vi "PAM icListen CC AV.vi"(4 "TCP IDs In":T2, 5 "Acq In":T1, 6 "icListen #":i32=1, 7 "Enabled":bool) -> (0 "TCP IDs Out":T2, 1 "Acq Out":T1, 3 "Stop":bool)   [LabVIEW 2020]
uses:
  icListen 1 Reset.vi
  icListen 1 Initialized.vi
  icListen 1 Connected.vi
  icListen 2 Reset.vi
  icListen 2 Initialized.vi
  icListen 2 Connected.vi
  icListen 3 Reset.vi
  icListen 3 Initialized.vi
  icListen 3 Connected.vi
  icListen 4 Reset.vi
  icListen 4 Initialized.vi
  icListen 4 Connected.vi
  icListen 1 Synchronization.vi
  icListen 1 Response.vi
  icListen 1 Metadata.vi
  icListen 2 Synchronization.vi
  icListen 2 Response.vi
  icListen 2 Metadata.vi
  icListen 3 Synchronization.vi
  icListen 3 Response.vi
  icListen 3 Metadata.vi
  icListen 4 Synchronization.vi
  icListen 4 Response.vi
  icListen 4 Metadata.vi
  PAM Array Buffer Size.vi
  icListen 1 Saving.vi
  icListen 2 Saving.vi
  icListen 3 Saving.vi
  icListen 4 Saving.vi
  icListen 1 Serial Number.vi
  icListen 2 Serial Number.vi
  icListen 3 Serial Number.vi
  icListen 4 Serial Number.vi
  PAM Library.lvlib
panel:
  out "Error Out":errorcluster
  out "Error Out":errorcluster
  out "Error Out":errorcluster
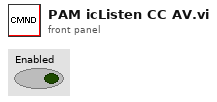
[diagram p1: front panel]
types:
  T1 = cluster{"State":enum16{"Align with Stream", "Read Header Byte", "Read Data Header", "Read Event Header", "Read Notification", "Read Data"}, "Sample Count":i32, "Timestamp":u64, "Payload":u16, "Repeated Error":i32, "Header Byte":string}
  T2 = cluster{"CC Id":refnum<k5>, "Waveform ID":refnum<k5>, "Spectrum ID":refnum<k5>, "Other Data ID":refnum<k5>}
  T3 = cluster{"System Time Status":u8, "Sync Status":u8, "PPS Count":u32, "Sync Offset":u32}
  T4 = cluster{"Date":string, "Time":string, "Temperature":dbl, "Humidity":dbl, "Battery Charge":i32}
  T5 = cluster{"default (0 U32) 2":i16, "default (0 U32)":i32, "unsigned 64bit integer":u64}
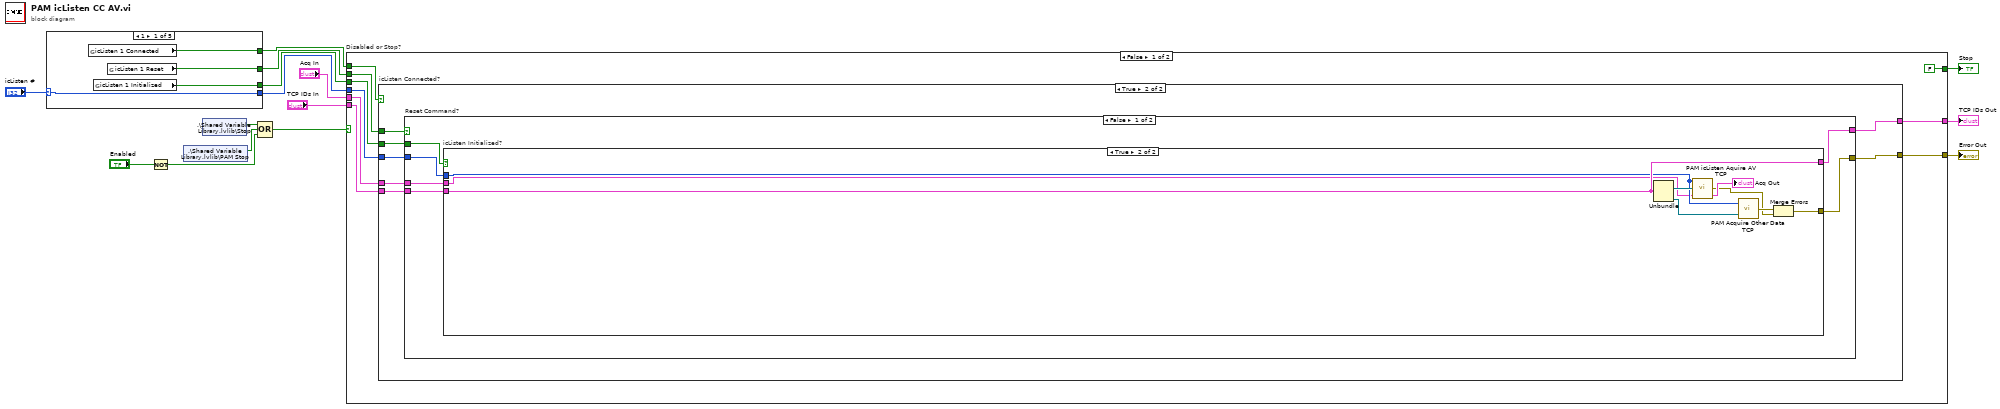
[diagram p0: block diagram]
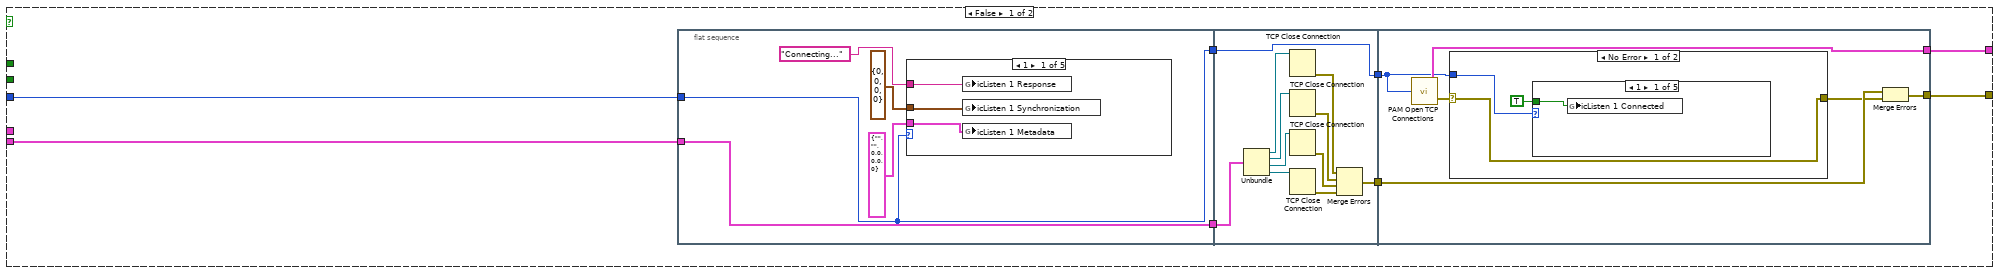
[diagram p2: hidden frame]
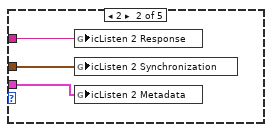
[diagram p3: hidden frame]
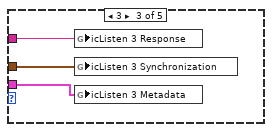
[diagram p4: hidden frame]
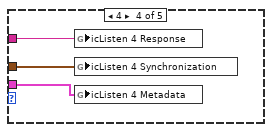
[diagram p5: hidden frame]
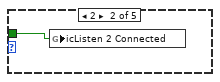
[diagram p7: hidden frame]
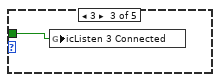
[diagram p8: hidden frame]
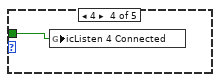
[diagram p9: hidden frame]
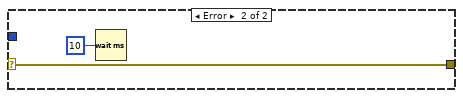
[diagram p11: hidden frame]
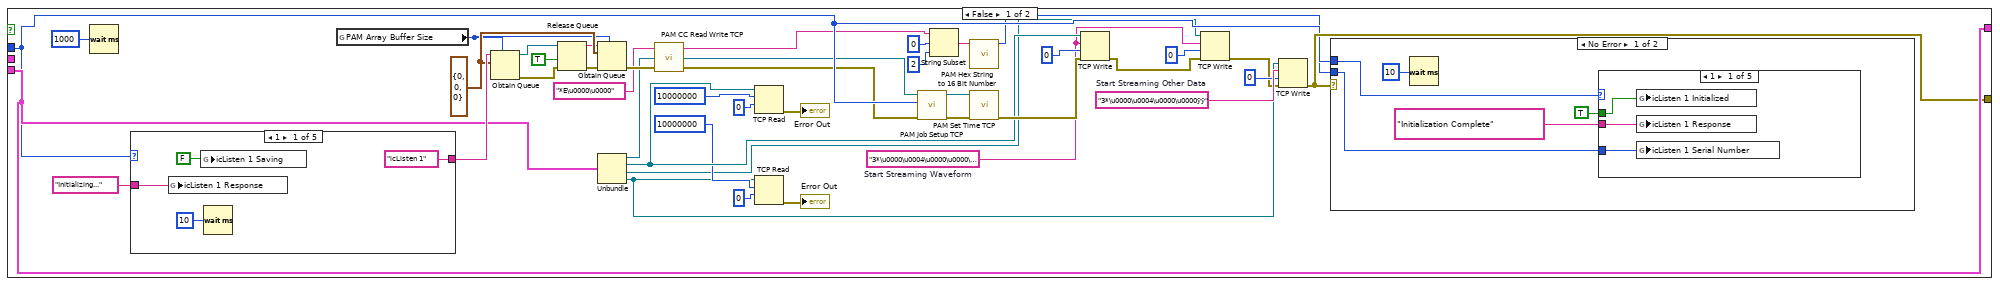
[diagram p12: hidden frame]
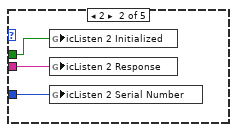
[diagram p13: hidden frame]
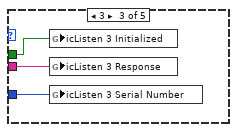
[diagram p14: hidden frame]
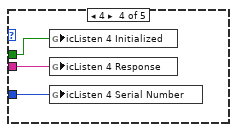
[diagram p15: hidden frame]
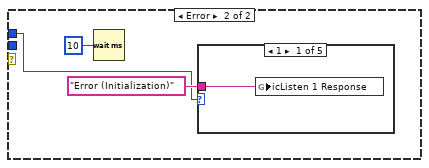
[diagram p17: hidden frame]
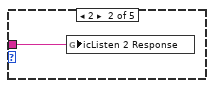
[diagram p18: hidden frame]
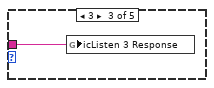
[diagram p19: hidden frame]
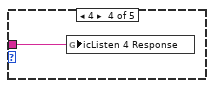
[diagram p20: hidden frame]
diagram:
  n1 = case shown="1" "icListen #" {
    selector: "icListen #" -> [w17 w20 w24 w28 _]
    tunnel: [w19 w23 w27 w31 _] -> w13
    tunnel: [w16 w21 w25 w29 _] -> w15
    tunnel: [w18 w22 w26 w30 _] -> w14
    tunnel: [w17 w20 w24 w28 0 ("icListen #")] -> w6
    frame 1 {
      n2 = global read "icListen 1 Connected.vi" "icListen 1 Connected"() -> (w16:bool)
      n3 = global read "icListen 1 Initialized.vi" "icListen 1 Initialized"() -> (w18:bool)
      n4 = global read "icListen 1 Reset.vi" "icListen 1 Reset"() -> (w19:bool)
    }
    frame 2 {
      n5 = global read "icListen 2 Connected.vi" "icListen 2 Connected"() -> (w21:bool)
      n6 = global read "icListen 2 Initialized.vi" "icListen 2 Initialized"() -> (w22:bool)
      n7 = global read "icListen 2 Reset.vi" "icListen 2 Reset"() -> (w23:bool)
    }
    frame 3 {
      n8 = global read "icListen 3 Connected.vi" "icListen 3 Connected"() -> (w25:bool)
      n9 = global read "icListen 3 Initialized.vi" "icListen 3 Initialized"() -> (w26:bool)
      n10 = global read "icListen 3 Reset.vi" "icListen 3 Reset"() -> (w27:bool)
    }
    frame 4 {
      n11 = global read "icListen 4 Connected.vi" "icListen 4 Connected"() -> (w29:bool)
      n12 = global read "icListen 4 Initialized.vi" "icListen 4 Initialized"() -> (w30:bool)
      n13 = global read "icListen 4 Reset.vi" "icListen 4 Reset"() -> (w31:bool)
    }
    frame 5, Default {
    }
  }
  n14 = Not(x="Enabled") -> (.not. x?=w1:bool)
  n15 = shared-variable ".\\Shared Variable Library.lvlib\\PAM Stop"() -> (w4:bool)  [unwired: 1 in, 1 out]
  n16 = shared-variable ".\\Shared Variable Library.lvlib\\Stop"() -> (w5:bool)  [unwired: 1 in, 1 out]
  n17 = Compound Arithmetic op=OR(w5, w4, w1) -> (w3:bool)
  n18 = case "Disabled or Stop?" shown="False" w3 {
    tunnel: w6 -> [w41 w240]
    tunnel: w15 -> [w40 _]
    tunnel: w14 -> [w39 _]
    tunnel: w13 -> [w38 _]
    tunnel: [FALSE w218] -> w12
    tunnel: [w36 w221] -> w10
    tunnel: "Acq In" -> [w35 _]
    tunnel: [w34 _] -> w9
    tunnel: "TCP IDs In" -> [w33 w231]
    frame False {
      n19 = case "icListen Connected?" shown="True" w40 {
        tunnel: w39 -> [_ w99]
        tunnel: w38 -> [_ w98]
        tunnel: [w47 w97] -> w36
        tunnel: w35 -> [_ w96]
        tunnel: w41 -> [w44 w95]
        tunnel: [w46 w93] -> w34
        tunnel: w33 -> [w49 w94]
        frame False {
          n20 = flat-sequence {
            tunnel: w49 -> [w54]
            tunnel: [w54] -> w45
            tunnel: w44 -> [w50]
            tunnel: [w50] -> w42
            tunnel: [w68] -> w48
            tunnel: w45 -> [w69]
            tunnel: [w67] -> w43
            tunnel: w42 -> [w67]
            tunnel: w48 -> [w82]
            tunnel: [w80] -> w47
            tunnel: [w79] -> w46
            tunnel: w43 -> [w78]
            frame #0 {
              n21 = case shown="1" w50 {
                tunnel: T4 {"Date"="", "Time"="", "Temperature"=0.0, "Humidity"=0.0, "Battery Charge"=0} ("icListen 1 Metadata") -> [w57 w60 w63 w65 _]
                tunnel: "Connecting..." ("icListen 2 Response 2") -> [w56 w59 w62 w66 _]
                tunnel: T3 {"System Time Status"=0, "Sync Status"=0, "PPS Count"=0, "Sync Offset"=0} ("icListen 4 Synchronization") -> [w55 w58 w61 w64 _]
                frame 1 {
                  n22 = global write "icListen 1 Response.vi" "icListen 1 Response"(w56) -> ()
                  n23 = global write "icListen 1 Synchronization.vi" "icListen 1 Synchronization"(w55) -> ()
                  n24 = global write "icListen 1 Metadata.vi" "icListen 1 Metadata"(w57) -> ()
                }
                frame 2 {
                  n25 = global write "icListen 2 Response.vi" "icListen 2 Response"(w59) -> ()
                  n26 = global write "icListen 2 Synchronization.vi" "icListen 2 Synchronization"(w58) -> ()
                  n27 = global write "icListen 2 Metadata.vi" "icListen 2 Metadata"(w60) -> ()
                }
                frame 3 {
                  n28 = global write "icListen 3 Response.vi" "icListen 3 Response"(w62) -> ()
                  n29 = global write "icListen 3 Synchronization.vi" "icListen 3 Synchronization"(w61) -> ()
                  n30 = global write "icListen 3 Metadata.vi" "icListen 3 Metadata"(w63) -> ()
                }
                frame 4 {
                  n31 = global write "icListen 4 Response.vi" "icListen 4 Response"(w66) -> ()
                  n32 = global write "icListen 4 Synchronization.vi" "icListen 4 Synchronization"(w64) -> ()
                  n33 = global write "icListen 4 Metadata.vi" "icListen 4 Metadata"(w65) -> ()
                }
                frame 5, Default {
                }
              }
            }
            frame #1 {
              n34 = Unbundle(w69) -> ("CC Id"=w74:refnum<k5>, "Waveform ID"=w75:refnum<k5>, "Spectrum ID"=w76:refnum<k5>, "Other Data ID"=w77:refnum<k5>)
              n35 = TCP Close Connection(connection ID=w74) -> (error out=w70:errorcluster)  [unwired: 2 in, 1 out]
              n36 = TCP Close Connection(connection ID=w75) -> (error out=w71:errorcluster)  [unwired: 2 in, 1 out]
              n37 = TCP Close Connection(connection ID=w76) -> (error out=w72:errorcluster)  [unwired: 2 in, 1 out]
              n38 = TCP Close Connection(connection ID=w77) -> (error out=w73:errorcluster)  [unwired: 2 in, 1 out]
              n39 = Merge Errors(w70, w71, w72, w73) -> (w68:errorcluster)
            }
            frame #2 {
              n40 = call "PAM Open TCP Connections.vi"("icListen #"=w78) -> ("TCP IDs"=w79:T2, "Error Out"=w83:errorcluster)
              n41 = case shown="No Error" w83 {
                selector: w83 -> [w85 w92]
                tunnel: [w85 w92] -> w81
                tunnel: w78 -> [w84 _]
                frame No Error {
                  n42 = case shown="1" w84 {
                    tunnel: TRUE -> [w87 w88 w89 w90 _]
                    frame 1 {
                      n43 = global write "icListen 1 Connected.vi" "icListen 1 Connected"(w87) -> ()
                    }
                    frame 2 {
                      n44 = global write "icListen 2 Connected.vi" "icListen 2 Connected"(w88) -> ()
                    }
                    frame 3 {
                      n45 = global write "icListen 3 Connected.vi" "icListen 3 Connected"(w89) -> ()
                    }
                    frame 4 {
                      n46 = global write "icListen 4 Connected.vi" "icListen 4 Connected"(w90) -> ()
                    }
                    frame 5, Default {
                    }
                  }
                }
                frame Error {
                  n47 = Wait (ms)(milliseconds to wait=u32 10) -> ()  [unwired: 1 out]
                }
              }
              n48 = Merge Errors(w82, w81) -> (w80:errorcluster)
            }
          }
        }
        frame True {
          n49 = case "Reset Command?" shown="False" w98 {
            tunnel: w99 -> [w105 _]
            tunnel: [w104 w201] -> w97
            tunnel: w96 -> [w103 _]
            tunnel: w95 -> [w102 w197]
            tunnel: w94 -> [w101 w199]
            tunnel: [w100 _] -> w93
            frame False {
              # "Reset False"
              n50 = case "icListen Initialized?" shown="True" w105 {
                tunnel: [w126 w188] -> w104
                tunnel: w103 -> [_ w192]
                tunnel: w102 -> [w122 w194]
                tunnel: w101 -> [w135 w195]
                tunnel: [w135 w195] -> w100
                frame False {
                  w137 = "3*\u0000\u0004\u0000\u0000ÿÿ"  # Start Streaming Other Data
                  w140 = T5 {"default (0 U32) 2"=0, "default (0 U32)"=0, "unsigned 64bit integer"=0} ("output cluster")
                  w120 = "3*\u0000\u0004\u0000\u0000\u0000\u0000"  # Start Streaming Waveform
                  n51 = Wait (ms)(milliseconds to wait=u32 1000) -> ()  [unwired: 1 out]
                  n52 = case shown="1" w122 {
                    tunnel: "Initializing..." ("Response") -> [w175 w179 w183 w187 _]
                    tunnel: ["icListen 1" ("name (unnamed)") "icListen 2" ("name (unnamed)") "icListen 3" ("name (unnamed)") "icListen 4" ("name (unnamed)") _] -> w144
                    frame 1 {
                      n53 = global write "icListen 1 Response.vi" "icListen 1 Response"(w175) -> ()
                      n54 = global write "icListen 1 Saving.vi" "icListen 1 Saving"(FALSE ("icListen 1 Saving")) -> ()
                      n55 = Wait (ms)(milliseconds to wait=u32 10) -> ()  [unwired: 1 out]
                    }
                    frame 2 {
                      n56 = global write "icListen 2 Response.vi" "icListen 2 Response"(w179) -> ()
                      n57 = global write "icListen 2 Saving.vi" "icListen 2 Saving"(FALSE ("icListen 2 Saving")) -> ()
                      n58 = Wait (ms)(milliseconds to wait=u32 10) -> ()  [unwired: 1 out]
                    }
                    frame 3 {
                      n59 = global write "icListen 3 Response.vi" "icListen 3 Response"(w183) -> ()
                      n60 = global write "icListen 3 Saving.vi" "icListen 3 Saving"(FALSE ("icListen 3 Saving")) -> ()
                      n61 = Wait (ms)(milliseconds to wait=u32 10) -> ()  [unwired: 1 out]
                    }
                    frame 4 {
                      n62 = global write "icListen 4 Response.vi" "icListen 4 Response"(w187) -> ()
                      n63 = global write "icListen 4 Saving.vi" "icListen 4 Saving"(FALSE ("icListen 4 Saving")) -> ()
                      n64 = Wait (ms)(milliseconds to wait=u32 10) -> ()  [unwired: 1 out]
                    }
                    frame 5, Default {
                    }
                  }
                  n65 = global read "PAM Array Buffer Size.vi" "PAM Array Buffer Size"() -> (w123:i32)
                  n66 = Obtain Queue(max queue size (-1, unlimited)=w123, name (unnamed)=w144, element data type=w140) -> (queue out=w142:refnum<queue>, error out=w141:errorcluster)  [unwired: 2 in, 1 out]
                  n67 = Release Queue(queue=w142, force destroy? (F)=TRUE, error in (no error)=w141) -> (queue name=w138:string, error out=w139:errorcluster)  [unwired: 1 out]
                  n68 = Obtain Queue(max queue size (-1, unlimited)=w123, name (unnamed)=w138, element data type=w140, error in (no error)=w139) -> (error out=w115:errorcluster)  [unwired: 1 in, 2 out]
                  n69 = Unbundle(w135) -> ("CC Id"=w112:refnum<k5>, "Waveform ID"=w132:refnum<k5>, "Spectrum ID"=w121:refnum<k5>, "Other Data ID"=w127:refnum<k5>)
                  n70 = call "PAM CC Read Write TCP.vi"("Error In"=w115, "ID In"=w112, "Command"="*E\u0000\u0000") -> ("Error Out"=w114:errorcluster, "ID Out"=w111:refnum<k5>, "Response"=w110:string)
                  n71 = TCP Read(connection ID=w132, bytes to read=10000000, 9:0 ("timeout ms (25000)")) -> (error out=→"Error Out":errorcluster)  [unwired: 2 in, 2 out]
                  n72 = TCP Read(connection ID=w127, bytes to read=10000000, 9:0 ("timeout ms (25000)")) -> (error out=→"Error Out":errorcluster)  [unwired: 2 in, 2 out]
                  n73 = call "PAM Job Setup TCP.vi"("Error In"=w114, "icListen #"=w122, "ID In"=w111) -> ("Error Out"=w146:errorcluster, "ID Out"=w145:refnum<k5>)  [unwired: 5 in, 1 out]
                  n74 = String Subset(string=w110, offset (0)=0, length (rest)=2 ("length (rest)")) -> (substring=w107:string)
                  n75 = call "PAM Hex String to 16 Bit Number.vi"("Hex String"=w107) -> ("Unsigned 16 Bit"=w106:u16)  [unwired: 9 in, 1 out]
                  n76 = call "PAM Set Time TCP.vi"("Error In"=w146, "ID In"=w145) -> ("Error Out"=w136:errorcluster)  [unwired: 6 in, 2 out]
                  n77 = TCP Write(connection ID=w132, data in=w120, error in (no error)=w136, 9:0 ("timeout ms (25000)")) -> (error out=w118:errorcluster)  [unwired: 2 out]
                  n78 = TCP Write(connection ID=w121, data in=w120, error in (no error)=w118, 9:0 ("timeout ms (25000)")) -> (error out=w117:errorcluster)  [unwired: 2 out]
                  n79 = TCP Write(connection ID=w127, data in=w137, error in (no error)=w117, 9:0 ("timeout ms (25000)")) -> (error out=w126:errorcluster)  [unwired: 2 out]
                  n80 = case shown="No Error" w126 {
                    tunnel: w122 -> [w149 w165]
                    tunnel: w106 -> [w148 _]
                    frame No Error {
                      n81 = Wait (ms)(milliseconds to wait=u32 10) -> ()  [unwired: 1 out]
                      n82 = case shown="1" w149 {
                        tunnel: TRUE -> [w154 w157 w160 w163 _]
                        tunnel: "Initialization Complete" ("icListen 2 Response 2") -> [w155 w158 w161 w164 _]
                        tunnel: w148 -> [w153 w156 w159 w162 _]
                        frame 1 {
                          n83 = global write "icListen 1 Initialized.vi" "icListen 1 Initialized"(w154) -> ()
                          n84 = global write "icListen 1 Response.vi" "icListen 1 Response"(w155) -> ()
                          n85 = global write "icListen 1 Serial Number.vi" "icListen 1 Serial Number"(w153) -> ()
                        }
                        frame 2 {
                          n86 = global write "icListen 2 Initialized.vi" "icListen 2 Initialized"(w157) -> ()
                          n87 = global write "icListen 2 Response.vi" "icListen 2 Response"(w158) -> ()
                          n88 = global write "icListen 2 Serial Number.vi" "icListen 2 Serial Number"(w156) -> ()
                        }
                        frame 3 {
                          n89 = global write "icListen 3 Initialized.vi" "icListen 3 Initialized"(w160) -> ()
                          n90 = global write "icListen 3 Response.vi" "icListen 3 Response"(w161) -> ()
                          n91 = global write "icListen 3 Serial Number.vi" "icListen 3 Serial Number"(w159) -> ()
                        }
                        frame 4 {
                          n92 = global write "icListen 4 Initialized.vi" "icListen 4 Initialized"(w163) -> ()
                          n93 = global write "icListen 4 Response.vi" "icListen 4 Response"(w164) -> ()
                          n94 = global write "icListen 4 Serial Number.vi" "icListen 4 Serial Number"(w162) -> ()
                        }
                        frame 5, Default {
                        }
                      }
                    }
                    frame Error {
                      n95 = Wait (ms)(milliseconds to wait=u32 10) -> ()  [unwired: 1 out]
                      n96 = case shown="1" w165 {
                        tunnel: "Error (Initialization)" ("icListen 2 Response 2") -> [w168 w169 w170 w171 _]
                        frame 1 {
                          n97 = global write "icListen 1 Response.vi" "icListen 1 Response"(w168) -> ()
                        }
                        frame 2 {
                          n98 = global write "icListen 2 Response.vi" "icListen 2 Response"(w169) -> ()
                        }
                        frame 3 {
                          n99 = global write "icListen 3 Response.vi" "icListen 3 Response"(w170) -> ()
                        }
                        frame 4 {
                          n100 = global write "icListen 4 Response.vi" "icListen 4 Response"(w171) -> ()
                        }
                        frame 5, Default {
                        }
                      }
                    }
                  }
                }
                frame True {
                  n101 = Unbundle(w195) -> ("Waveform ID"=w196:refnum<k5>, "Other Data ID"=w193:refnum<k5>)  [unwired: 2 out]
                  n102 = call "PAM icListen Aquire AV TCP.vi"("Acq In"=w192, "ID In"=w196, "icListen #"=w194) -> ("Acq Out"=→"Acq Out":T1, "Error Out"=w189:errorcluster)  [unwired: 1 in]
                  n103 = call "PAM Acquire Other Data TCP.vi"("Other Data ID"=w193, "icListen #"=w194) -> ("Error Out"=w190:errorcluster)
                  n104 = Merge Errors(w190, w189) -> (w188:errorcluster)
                }
              }
            }
            frame True {
              w205 = "*Y\u0000\u0000"  # Reset Command
              # "Reset True"
              n105 = Wait (ms)(milliseconds to wait=u32 10) -> ()  [unwired: 1 out]
              n106 = case shown="1" w197 {
                tunnel: FALSE -> [w206 w210 w213 w216 _]
                tunnel: "Resetting icListen" ("Response") -> [w208 w211 w214 w217 _]
                tunnel: T3 {"System Time Status"=0, "Sync Status"=0, "PPS Count"=0, "Sync Offset"=0} ("icListen 4 Synchronization") -> [w207 w209 w212 w215 _]
                frame 1 {
                  n107 = global write "icListen 1 Synchronization.vi" "icListen 1 Synchronization"(w207) -> ()
                  n108 = global write "icListen 1 Response.vi" "icListen 1 Response"(w208) -> ()
                  n109 = global write "icListen 1 Connected.vi" "icListen 1 Connected"(w206) -> ()
                  n110 = global write "icListen 1 Initialized.vi" "icListen 1 Initialized"(w206) -> ()
                  n111 = global write "icListen 1 Reset.vi" "icListen 1 Reset"(w206) -> ()
                }
                frame 2 {
                  n112 = global write "icListen 2 Synchronization.vi" "icListen 2 Synchronization"(w209) -> ()
                  n113 = global write "icListen 2 Response.vi" "icListen 2 Response"(w211) -> ()
                  n114 = global write "icListen 2 Reset.vi" "icListen 2 Reset"(w210) -> ()
                  n115 = global write "icListen 2 Connected.vi" "icListen 2 Connected"(w210) -> ()
                  n116 = global write "icListen 2 Initialized.vi" "icListen 2 Initialized"(w210) -> ()
                }
                frame 3 {
                  n117 = global write "icListen 3 Synchronization.vi" "icListen 3 Synchronization"(w212) -> ()
                  n118 = global write "icListen 3 Response.vi" "icListen 3 Response"(w214) -> ()
                  n119 = global write "icListen 3 Reset.vi" "icListen 3 Reset"(w213) -> ()
                  n120 = global write "icListen 3 Connected.vi" "icListen 3 Connected"(w213) -> ()
                  n121 = global write "icListen 3 Initialized.vi" "icListen 3 Initialized"(w213) -> ()
                }
                frame 4 {
                  n122 = global write "icListen 4 Synchronization.vi" "icListen 4 Synchronization"(w215) -> ()
                  n123 = global write "icListen 4 Response.vi" "icListen 4 Response"(w217) -> ()
                  n124 = global write "icListen 4 Reset.vi" "icListen 4 Reset"(w216) -> ()
                  n125 = global write "icListen 4 Connected.vi" "icListen 4 Connected"(w216) -> ()
                  n126 = global write "icListen 4 Initialized.vi" "icListen 4 Initialized"(w216) -> ()
                }
                frame 5, Default {
                }
              }
              n127 = Unbundle(w199) -> ("CC Id"=w198:refnum<k5>)  [unwired: 3 out]
              n128 = call "PAM CC Read Write TCP.vi"("ID In"=w198, "Command"=w205) -> ("Error Out"=w201:errorcluster)  [unwired: 1 in, 2 out]
            }
          }
        }
      }
    }
    frame True {
      w229 = "4*\u0000\u0000"  # Stop Streaming
      w237 = "4*\u0000\u0000"  # Stop Streaming
      w239 = "4*\u0000\u0000"  # Stop Streaming
      n129 = case shown="1" w240 {
        tunnel: FALSE -> [w245 w251 w255 w259 _]
        tunnel: "Disabled" ("icListen 2 Response 2") -> [w248 w252 w256 w260 _]
        tunnel: T4 {"Date"="", "Time"="", "Temperature"=0.0, "Humidity"=0.0, "Battery Charge"=0} ("icListen 1 Metadata") -> [w247 w250 w254 w258 _]
        tunnel: T3 {"System Time Status"=0, "Sync Status"=0, "PPS Count"=0, "Sync Offset"=0} ("Synchronization") -> [w246 w249 w253 w257 _]
        frame 1 {
          n130 = global write "icListen 1 Response.vi" "icListen 1 Response"(w248) -> ()
          n131 = global write "icListen 1 Initialized.vi" "icListen 1 Initialized"(w245) -> ()
          n132 = global write "icListen 1 Connected.vi" "icListen 1 Connected"(w245) -> ()
          n133 = global write "icListen 1 Metadata.vi" "icListen 1 Metadata"(w247) -> ()
          n134 = global write "icListen 1 Synchronization.vi" "icListen 1 Synchronization"(w246) -> ()
        }
        frame 2 {
          n135 = global write "icListen 2 Response.vi" "icListen 2 Response"(w252) -> ()
          n136 = global write "icListen 2 Initialized.vi" "icListen 2 Initialized"(w251) -> ()
          n137 = global write "icListen 2 Connected.vi" "icListen 2 Connected"(w251) -> ()
          n138 = global write "icListen 2 Metadata.vi" "icListen 2 Metadata"(w250) -> ()
          n139 = global write "icListen 2 Synchronization.vi" "icListen 2 Synchronization"(w249) -> ()
        }
        frame 3 {
          n140 = global write "icListen 3 Response.vi" "icListen 3 Response"(w256) -> ()
          n141 = global write "icListen 3 Initialized.vi" "icListen 3 Initialized"(w255) -> ()
          n142 = global write "icListen 3 Connected.vi" "icListen 3 Connected"(w255) -> ()
          n143 = global write "icListen 3 Metadata.vi" "icListen 3 Metadata"(w254) -> ()
          n144 = global write "icListen 3 Synchronization.vi" "icListen 3 Synchronization"(w253) -> ()
        }
        frame 4 {
          n145 = global write "icListen 4 Response.vi" "icListen 4 Response"(w260) -> ()
          n146 = global write "icListen 4 Initialized.vi" "icListen 4 Initialized"(w259) -> ()
          n147 = global write "icListen 4 Connected.vi" "icListen 4 Connected"(w259) -> ()
          n148 = global write "icListen 4 Metadata.vi" "icListen 4 Metadata"(w258) -> ()
          n149 = global write "icListen 4 Synchronization.vi" "icListen 4 Synchronization"(w257) -> ()
        }
        frame 5, Default {
        }
      }
      n150 = Unbundle(w231) -> ("CC Id"=w230:refnum<k5>, "Waveform ID"=w227:refnum<k5>, "Spectrum ID"=w226:refnum<k5>, "Other Data ID"=w225:refnum<k5>)
      n151 = shared-variable ".\\Shared Variable Library.lvlib\\PAM Stop"() -> (w220:bool)  [unwired: 1 in, 1 out]
      n152 = TCP Write(connection ID=w227, data in=w237) -> (connection ID out=w236:refnum<k5>, error out=w224:errorcluster)  [unwired: 2 in, 1 out]
      n153 = TCP Write(connection ID=w226, data in=w239) -> (connection ID out=w238:refnum<k5>, error out=w223:errorcluster)  [unwired: 2 in, 1 out]
      n154 = TCP Write(connection ID=w225, data in=w229) -> (connection ID out=w228:refnum<k5>, error out=w222:errorcluster)  [unwired: 2 in, 1 out]
      n155 = shared-variable ".\\Shared Variable Library.lvlib\\Stop"() -> (w219:bool)  [unwired: 1 in, 1 out]
      n156 = TCP Close Connection(connection ID=w230) -> (error out=w232:errorcluster)  [unwired: 2 in, 1 out]
      n157 = TCP Close Connection(connection ID=w236) -> (error out=w234:errorcluster)  [unwired: 2 in, 1 out]
      n158 = TCP Close Connection(connection ID=w238) -> (error out=w233:errorcluster)  [unwired: 2 in, 1 out]
      n159 = TCP Close Connection(connection ID=w228) -> (error out=w235:errorcluster)  [unwired: 2 in, 1 out]
      n160 = Merge Errors(w235, w234, w233, w232, w224, w223, w222) -> (w221:errorcluster)
      n161 = Compound Arithmetic op=OR(w219, w220) -> (w218:bool)
    }
  }
  "Stop" <- w12
  "Error Out" <- w10
  "TCP IDs Out" <- w9
